vi "IncludeProjectLibrary_NotIncludeSubLibraries_WhitelistNotContainsSubLibrary.vi"(9 "file":path) -> (0 "error out":errorcluster)   [LabVIEW 2017, in "Whitelist.Tests.lvlib"]
uses:
  Whitelist.Tests.lvlib
  Whitelist/Whitelist.lvclass
  Assertion/Assertion.lvlib
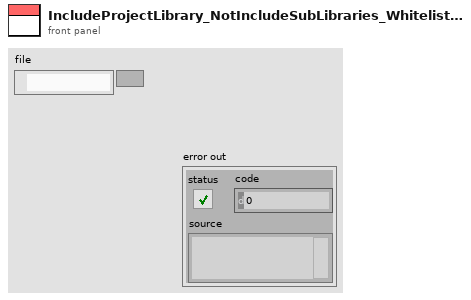
[diagram p1: front panel]
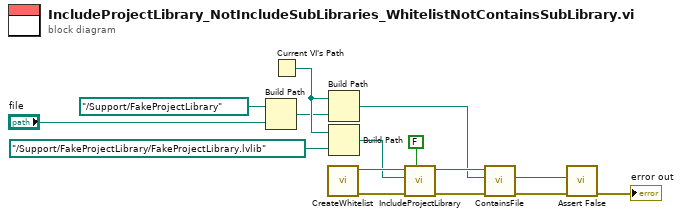
[diagram p0: block diagram]
diagram:
  n1 = Build Path(base path=path "../Support/FakeProjectLibrary", name or relative path="file") -> (appended path=w3:path)
  n2 = Current VI's Path() -> (path=w7:path)
  n3 = call "CreateWhitelist.vi"() -> ("error out"=w14:errorcluster, "Whitelist out"=w15:refnum<class "Whitelist.lvclass">)  [unwired: 10 in]
  n4 = Build Path(base path=w7, name or relative path=w3) -> (appended path=w6:path)
  n5 = Build Path(base path=w7, name or relative path=path "../Support/FakeProjectLibrary/FakeProjectLibrary.lvlib" ("relative_library_path")) -> (appended path=w8:path)
  n6 = call "IncludeProjectLibrary.vi"("Include Sub Libraries (T)"=FALSE, "error in (no error)"=w14, "Path"=w8, "Whitelist in"=w15) -> ("error out"=w12:errorcluster, "Whitelist out"=w13:refnum<class "Whitelist.lvclass">)  [unwired: 6 in]
  n7 = call "ContainsFile.vi"("error in (no error)"=w12, "Path"=w6, "Whitelist in"=w13) -> ("error out"=w11:errorcluster, "Is Whitelisted?"=w10:bool)  [unwired: 6 in, 1 out]
  n8 = call "Assert False.vi"("error in (no error)"=w11, "Condition"=w10) -> ("error out"=→"error out":errorcluster)  [unwired: 9 in]
